vi "zmq_endpoint_build.vi"(4 "error in":errorcluster, 5 "port":u16, 6 "address":string="127.0.0.1", 7 "protocol (tcp)":T1) -> (0 "error out":errorcluster, 1 "port out":u16, 3 "endpoint":string)   [LabVIEW 2020, in "zeromq.lvlib"]
doc: "Constructs a string that can be used as an \"endpoint\" for connect or bind operations from consistuent parts.\n\nIf <b>port</b> is 0, a random unused (ephemeral) port is selected."
uses:
  zeromq.lvlib
  endpoint_proto.ctl
panel:
  # "ØMQ"
  # "labview"
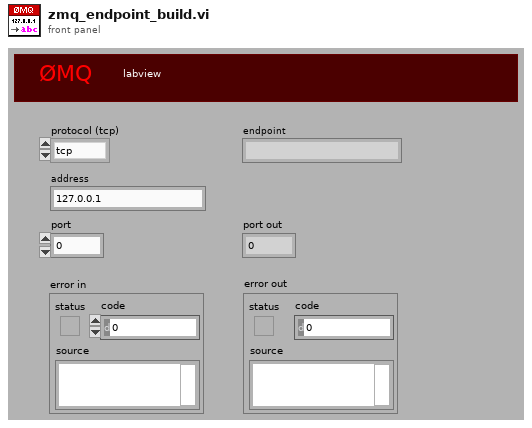
[diagram p1: front panel]
types:
  T1 = typedef "zeromq.lvlib/endpoint_proto.ctl" = enum16{"tcp", "inproc"}
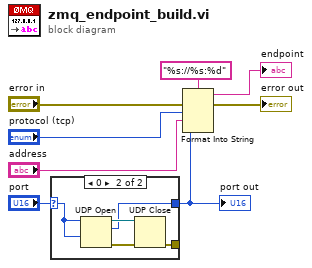
[diagram p0: block diagram]
diagram:
  n1 = case shown="0" "port" {
    selector: "port" -> [w9 w14]
    tunnel: [w9 w12] -> w1
    tunnel: [_ w10] -> _
    frame Default {
    }
    frame 0 {
      n2 = UDP Open(9:w14, 11:w14) -> (port=w13:refnum<k16>, 0:w11:errorcluster, 2:w12:u16)  [unwired: 3 in]
      n3 = UDP Close(connection ID=w13, 8:w11) -> (error out=w10:errorcluster)  [unwired: 1 out]
    }
  }
  "port out" <- w1
  n4 = Format Into String(format string="%s://%s:%d", error in="error in", "protocol (tcp)", "address", w1) -> (resulting string=→"endpoint":string, error out=→"error out":errorcluster)  [unwired: 1 in]
